vi "updateIntensityData.vi"(8 "new x":dbl, 9 "Images 2D":dbl[][][](array[numeric]), 10 "Image Intensity (initial)":dbl[][](array[numeric]), 11 "x-axis (initial)":dbl[](array[numeric])) -> (0 "x-axis (final = initial + new)":dbl[](array[numeric]), 1 "Added Image Intensity (I_new)":dbl[](array[numeric]), 2 "Image Intensity (final = I_initial + I_new)":dbl[][](array[numeric]), 3 "Image Intensity vs x":cluster{dbl[], dbl[]}[](array[cluster]))   [LabVIEW 2012]
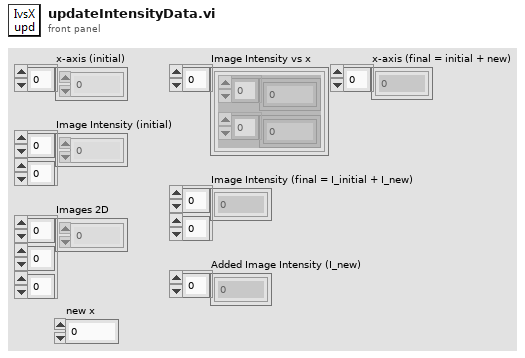
[diagram p1: front panel]
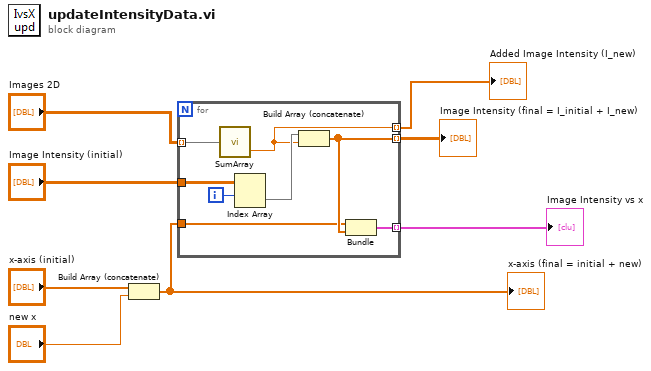
[diagram p0: block diagram]
diagram:
  n1 = Build Array (concatenate)("x-axis (initial)", "new x") -> (w1:dbl[])
  "x-axis (final = initial + new)" <- w1
  n2 = for {
    tunnel: "Images 2D" -> [w16] mode=indexing
    tunnel: w1 -> [w11]
    tunnel: "Image Intensity (initial)" -> [w14]
    tunnel: [w15] -> w7 mode=indexing
    tunnel: [w12] -> w6 mode=indexing
    tunnel: [w9] -> w8 mode=indexing
    i -> [w10]
    n3 = call "SumArray.vi"("Array"=w16) -> ("Average"=w9:dbl)  [unwired: 1 out]
    n4 = Index Array(array=w14, index (row)=w10) -> (element=w13:dbl[])  [unwired: 1 in]
    n5 = Build Array (concatenate)(w13, w9) -> (w12:dbl[])
    n6 = Bundle(w11, w12) -> (w15:cluster{dbl[], dbl[]})  [unwired: 1 in]
  }
  "Added Image Intensity (I_new)" <- w8
  "Image Intensity vs x" <- w7
  "Image Intensity (final = I_initial + I_new)" <- w6
